vi "Oscilloscope_tests.vi"() -> ()   [LabVIEW 2019]
doc: "This example shows how to configure multiple channels and acquire waveforms from multiple channels."
uses:
  <vilib>/Utility/error.llb/DialogType.ctl
  subVIs/SiPM_Tests_Global_Var.vi
  subVIs/Agilent_lib/Public/Configure/Trigger/Configure Trigger (Edge).vi
  subVIs/Agilent_lib/Agilent 2000 3000 X-Series.lvlib
panel:
  in  "Close Session":bool
  out "Meas Ind":bool
  in  "HP8116A":refnum<visa-resource-name>="GPIB0::16::INSTR" caption="Function Generator HP8116A"
  in  "Power supply Agilent E3631A":refnum<visa-resource-name>="GPIB0::5::INSTR"
  in  "x = y?":bool
  in  "Stop Button 2":bool
  in  "Free Run 2":bool
  in  "Frames to Run":dbl
  in  "Time to Run (s)":dbl
  in  "System Settings":bool
  in  "Load file to display":bool
  in  "Spectrum Only":bool
  in  "Stop Button":bool
  in  "Free Run":bool
  in  "Tab Control":enum32{"Energy Spectrum"}(tab)
  out "XY Graph":T1(graph) caption="Energy Spectrum"
  in  "Coincidence?":bool
  out "en_channels":bool[](array[boolean])
  in  "Trigger Source":T2(ring)
  in  "Input \nCoupling":T3(ring)=enum."DC Coupling"
  in  "Edge \nSlope":enum16{"Pos", "Neg", "Either", "Alt"}(ring)
  in  "Trigger Level (V)":dbl(knob)=0.003 min=-10.0 max=10.0 step=0.01 scale=0.0..5.0
  in  "EN 4":bool=TRUE
  in  "Ch 4 Vertical Scale":dbl(knob)=0.002 min=0.0 max=5.0 step=0.05 scale=0.0..5.0
  in  "CH 4  offset":dbl(knob)=0.006 min=-10.0 max=10.0 step=0.01 scale=0.0..10.0
  in  "Ch3 Vertical Scale":dbl(knob)=0.002 min=0.0 max=5.0 step=0.05 scale=0.0..5.0
  in  "CH 3  offset":dbl(knob)=0.006 min=-10.0 max=10.0 step=0.01 scale=0.0..10.0
  in  "EN 3":bool
  in  "EN 2":bool=TRUE
  in  "Ch 2 Vertical Scale":dbl(knob)=0.002 min=0.0 max=5.0 step=0.05 scale=0.0..5.0
  in  "CH 2  offset":dbl(knob)=0.006 min=-10.0 max=10.0 step=0.01 scale=0.0..10.0
  in  "Ch1 Vertical Scale":dbl(knob)=0.002 min=0.0 max=5.0 step=0.001 scale=0.0..5.0
  in  "CH 1  offset":dbl(knob)=0.006 min=-10.0 max=10.0 step=0.01 scale=0.0..10.0
  in  "EN":bool=TRUE
  in  "Agilent MSO-X 3104A \nOscilloscope":refnum<visa-resource-name>="USB0::0x0957::0x1780::MY56270584::INSTR"
  out "Scope":waveform(dbl)[](graph)
  in  "Impedance":enum16{"1 MOhm", "50 Ohm"}(ring)=enum."50 Ohm"
  in  "Coupling":enum16{"AC", "DC"}(ring)=enum."DC"
  in  "Vertical Setting":enum16{"Vertical Scale", "Vertical Range"}(ring)
  in  "Vertical Range":dbl=40.0
  in  "Time per Division":dbl(knob)=1e-06 scale=0.0..1.0
  in  "Horizontal \nPosition":dbl(knob) scale=0.0..1.0
  in  "Ch1":u8=1 min=1 max=10 step=9
  in  "Ch2":u8=1 min=1 max=10 step=9
  in  "Ch3":u8=1 min=1 max=10 step=9
  in  "Ch4":u8=1 min=1 max=10 step=9
  in  "Bin Min (V)":dbl format="%#_6p"
  in  "Bin Max (V)":dbl=0.026 format="%#_6p"
  out "Pulser":bool
  out "Bias":bool
  out "Power":bool
  out "Scope":bool
  out "Session Log":string
  in  "Read Temperature":bool
  out "Celcius":dbl(slide) scale=0.0..30.0
  in  "Default?":bool=TRUE
  out "Time (s)":dbl format="%.2f"
  in  "Save Results?":bool
  in  "Temperature":string
  in  "Settings Button":bool
  in  "Results Directory":path=path "C:/Users/johnk/Desktop/ESA_Scintillator_Data"
  out "Frames Recorded":i32
  in  "Measurement":string
  in  "File Name":string="1"
  in  "Enable\nVernier":bool
  in  "Enable \nREF \nBNC":bool
  in  "Time Base Type":i32(ring) items=["Main", "Window", "XY", "Roll"]
  # "NCSR  DEMOKRITOS\nInstitute of Nuclear and Particle Physics\nDetectors Instrumentation Laboratory"
  # "CFD Scope Tests"
  # "Record Waveform"
  # "Run Noise Tests"
  # "Probe Attenuation"
  # "RIGOL DG4102 \nFunction Generator"
  # "Histogram Bin"
  # "CH1\n30V/3A"
  # "CH2\n(HV)"
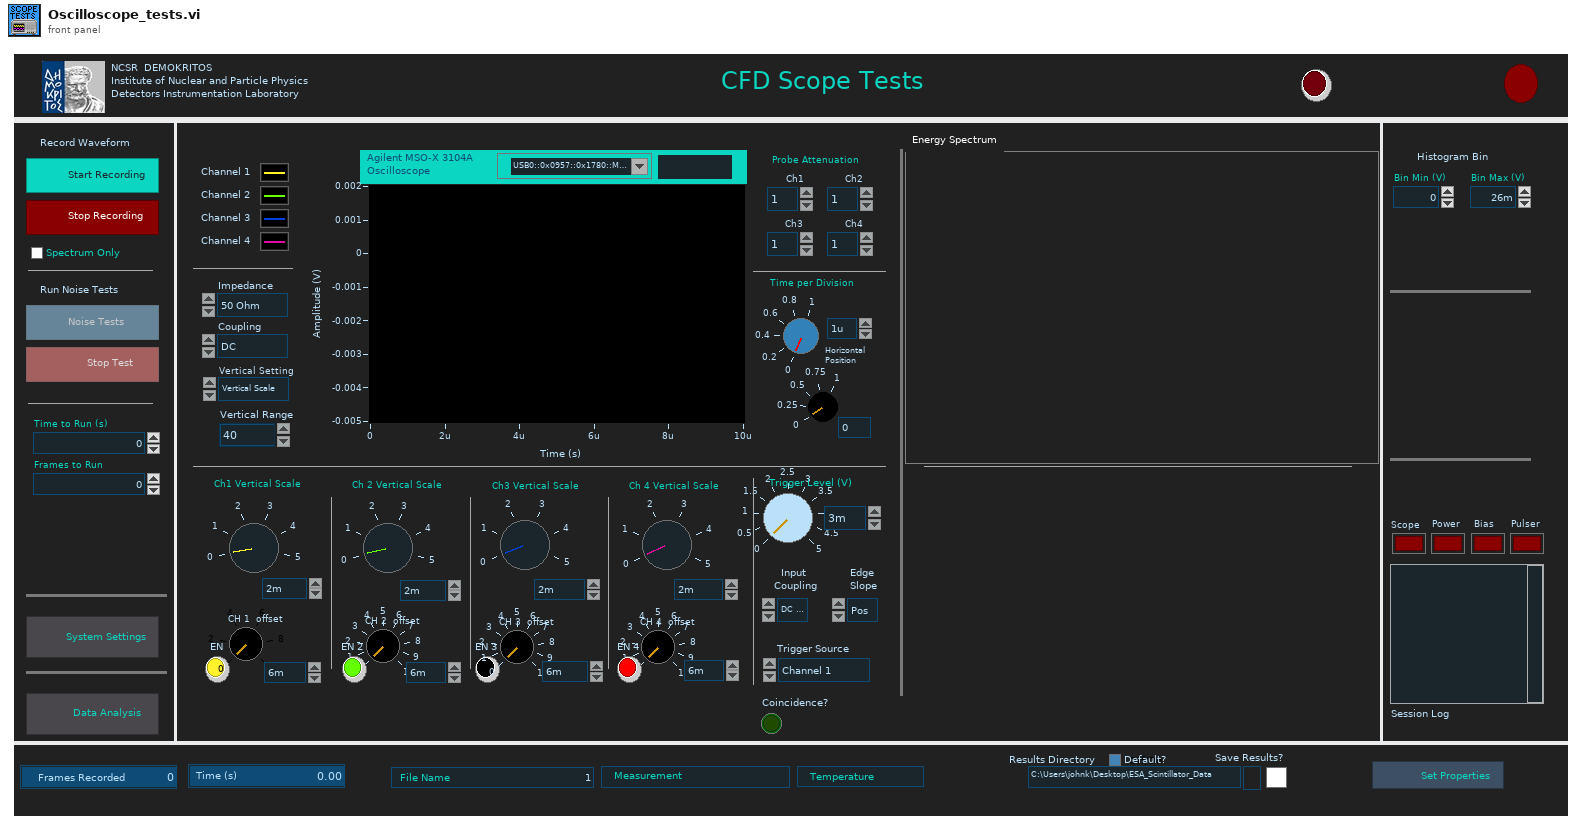
[diagram p1: front panel]
types:
  T1 = cluster{"X Values":dbl[], "Histogram: h(x)":i32[]}[]
  T2 = enum16{"Channel 1", "Channel 2", "Channel 3", "Channel 4", "D0", "D1", "D2", "D3", "D4", "D5", "D6", "D7", "D8", "D9", "D10", "D11", "D12", "D13", "D14", "D15", "External", "Power Line", "Waveform Generator"}
  T3 = enum16{"AC Coupling", "DC Coupling", "Low Frequency Reject"}
  T4 = typedef "DialogType.ctl" = u16
  T5 = cluster{"error":bool, "code":i32, "source":string}
  T6 = enum16{"big-endian, network order", "native, host order", "little-endian"}
  T7 = enum16{"open", "open or create", "create or replace", "create", "open (read-only)"}
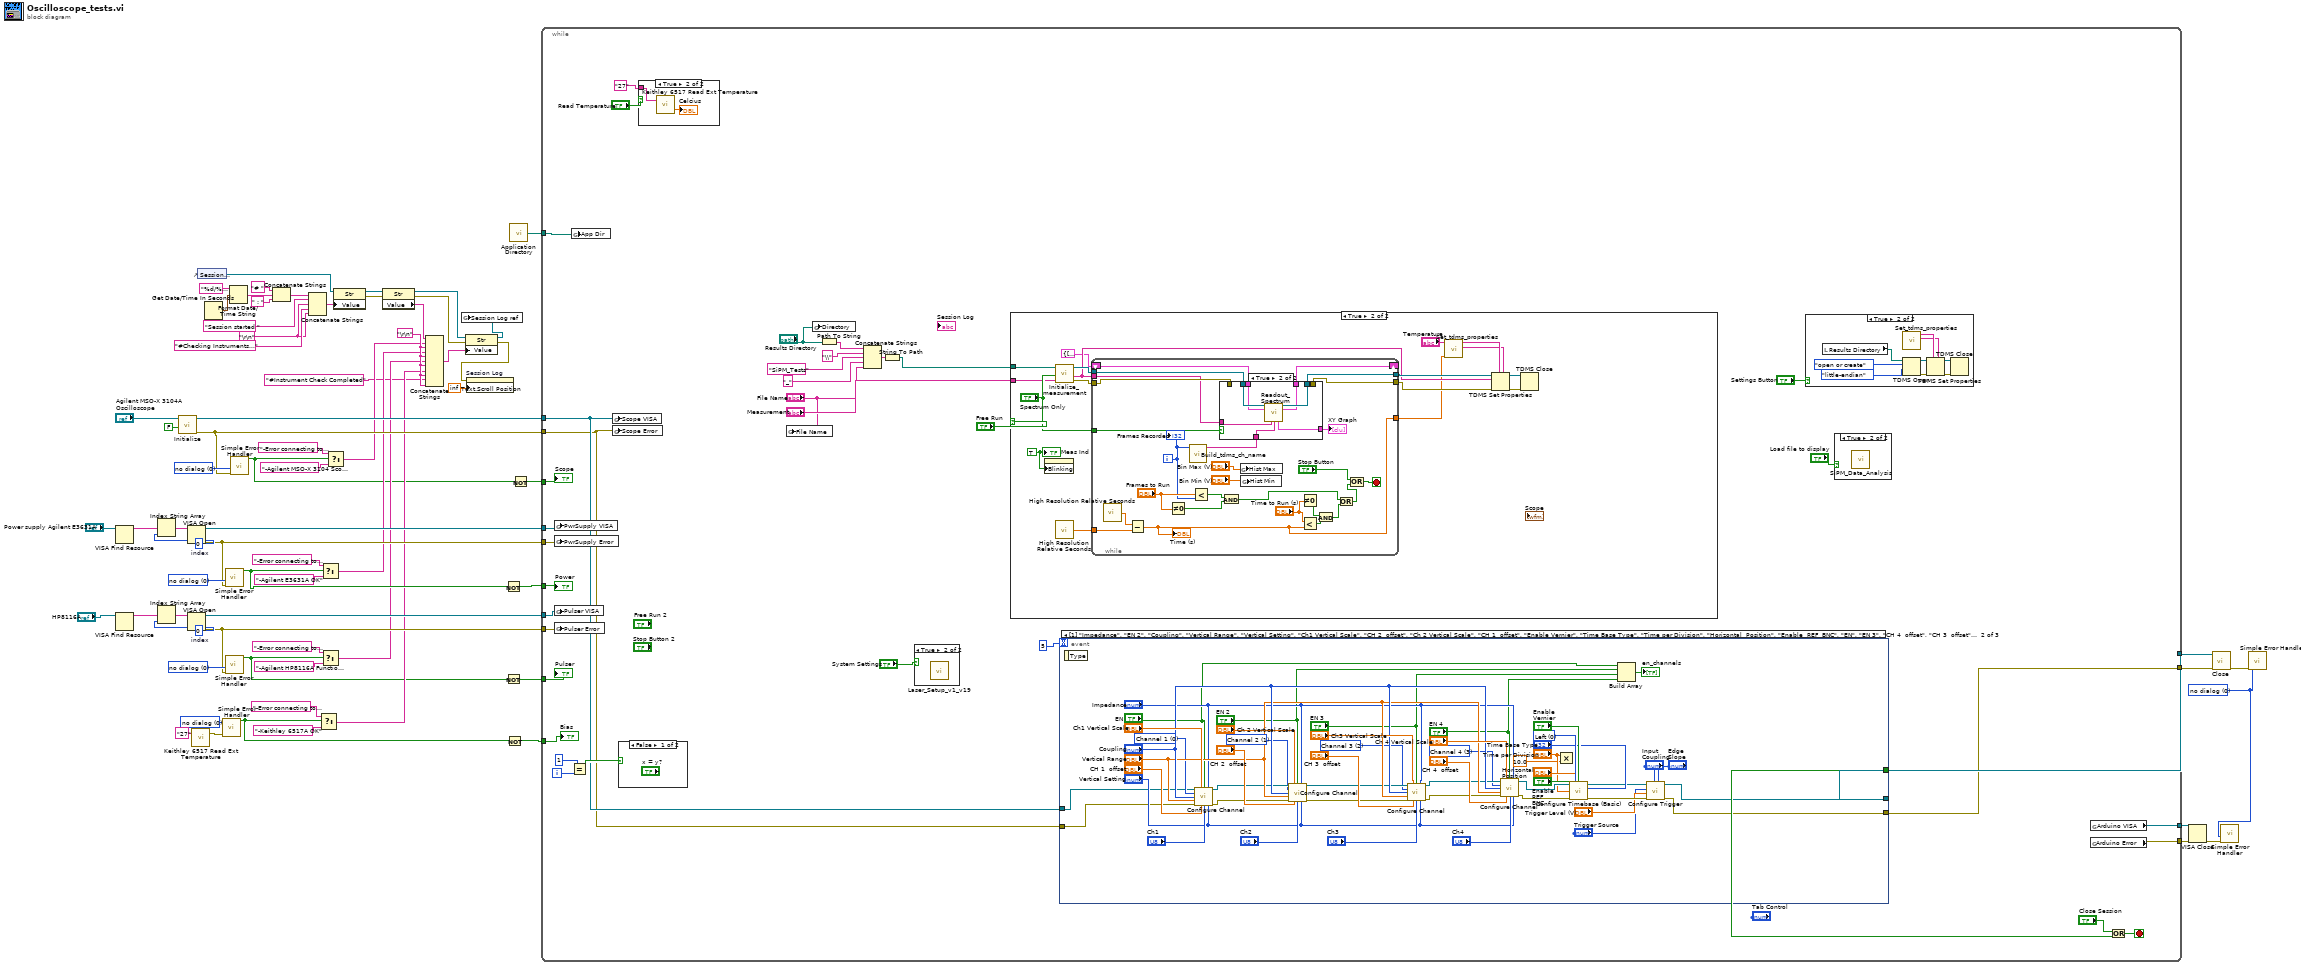
[diagram p0: block diagram]
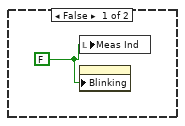
[diagram p4: hidden frame]
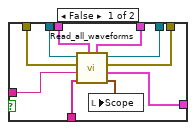
[diagram p5: hidden frame]
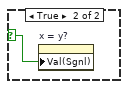
[diagram p6: hidden frame]
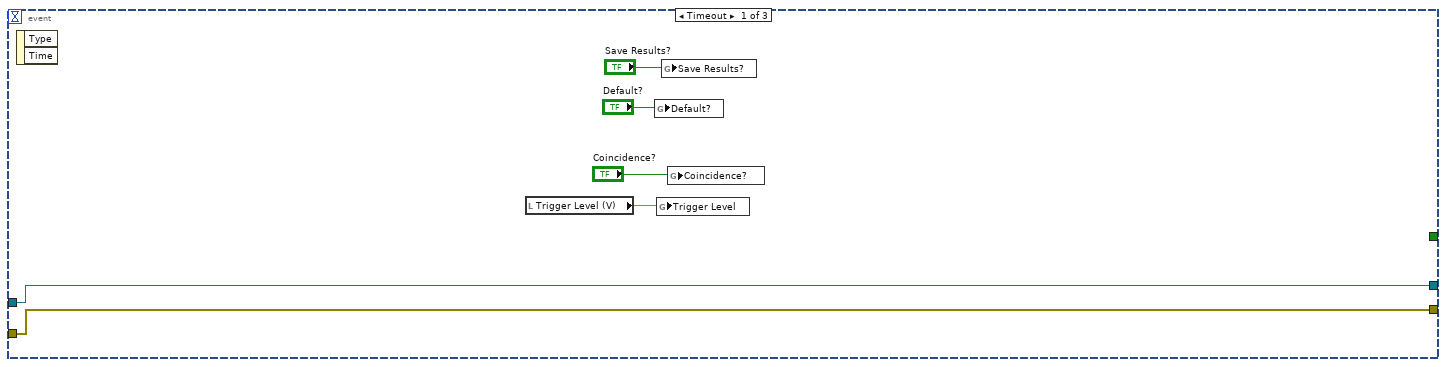
[diagram p9: hidden frame]
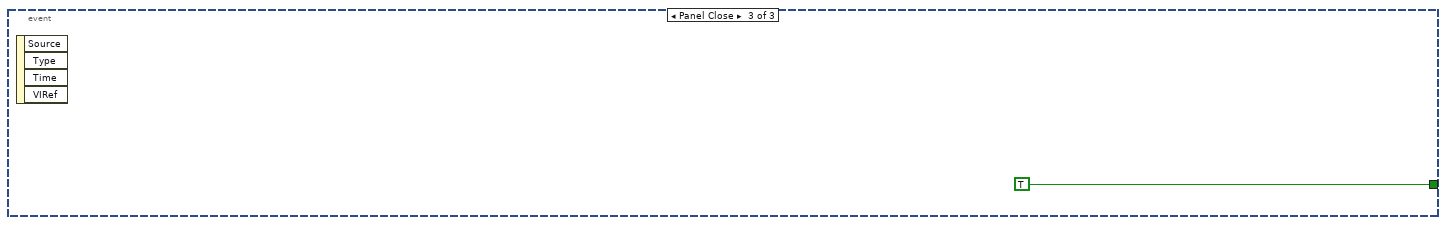
[diagram p10: hidden frame]
diagram:
  w1 = T4 0 items=["no dialog", "OK message", "continue or stop message", "OK message + warnings", "continue/stop + warnings"] ("type of dialog (OK msg:1)")
  w20 = T4 0 items=["no dialog", "OK message", "continue or stop message", "OK message + warnings", "continue/stop + warnings"] ("type of dialog (OK msg:1)")
  w31 = T4 0 items=["no dialog", "OK message", "continue or stop message", "OK message + warnings", "continue/stop + warnings"] ("type of dialog (OK msg:1)")
  w27 = 0  # index
  w36 = T4 0 items=["no dialog", "OK message", "continue or stop message", "OK message + warnings", "continue/stop + warnings"] ("type of dialog (OK msg:1)")
  w42 = 0  # index
  w48 = T4 0 items=["no dialog", "OK message", "continue or stop message", "OK message + warnings", "continue/stop + warnings"] ("type of dialog (OK msg:1)")
  w52 = "\r\n"
  w58 = "\r\n"
  w67 = FALSE ("ID Query (True)")
  n1 = VISA Find Resource(11:"Power supply Agilent E3631A") -> (3:w41:string[])  [unwired: 2 in, 2 out]
  n2 = VISA Find Resource(11:"HP8116A") -> (3:w28:string[])  [unwired: 2 in, 2 out]
  n3 = Index String Array(1:w42, 2:w41) -> (0:w39:string)  [unwired: 1 in]
  n4 = Index String Array(1:w27, 2:w28) -> (0:w29:string)  [unwired: 1 in]
  n5 = call "Initialize.vi"("Reset (True)"=w67, "ID Query (True)"=w67, "VISA resource name"="Agilent MSO-X 3104A \nOscilloscope") -> ("error out"=w47:errorcluster, "VISA resource name out"=w71:refnum<visa-resource-name>)  [unwired: 2 in, 5 out]
  n6 = VISA Open(VISA resource name=w39) -> (VISA resource name=w38:refnum<visa-resource-name>, error out=w35:errorcluster)  [unwired: 4 in]
  n7 = VISA Open(VISA resource name=w29) -> (VISA resource name=w25:refnum<visa-resource-name>, error out=w24:errorcluster)  [unwired: 4 in]
  n8 = call "Keithley 6517 Read Ext Temperature.vi"("GPIB address"="27") -> ("error out"=w21:T5)  [unwired: 1 in, 1 out]
  n9 = control-ref of="Session Log"() -> (w54:refnum<vi>)
  n10 = Get Date/Time In Seconds() -> (seconds since 1Jan1904=w64:timestamp)
  n11 = call <vilib>:"Simple Error Handler.vi"("type of dialog (OK msg:1)"=w20, "error in (no error)"=w21) -> ("error?"=w14:bool)  [unwired: 3 in, 4 out]
  n12 = call <vilib>:"Simple Error Handler.vi"("type of dialog (OK msg:1)"=w36, "error in (no error)"=w35) -> ("error?"=w33:bool)  [unwired: 3 in, 4 out]
  n13 = call <vilib>:"Simple Error Handler.vi"("type of dialog (OK msg:1)"=w31, "error in (no error)"=w24) -> ("error?"=w12:bool)  [unwired: 3 in, 4 out]
  n14 = Format Date/Time String(time format string (%c)="%d/%m/%y_%H:%M:%S", seconds (now)=w64) -> (date/time string=w62:string)  [unwired: 1 in]
  n15 = call <vilib>:"Simple Error Handler.vi"("type of dialog (OK msg:1)"=w48, "error in (no error)"=w47) -> ("error?"=w9:bool)  [unwired: 3 in, 4 out]
  n16 = Concatenate Strings("# " ("string"), w62, " : " ("string")) -> (w61:string)
  n17 = Concatenate Strings(w61, "Session started ", w58, "#Checking Instruments..." ("string"), w58) -> (w57:string)
  n18 = Select(t="-Error connecting to Keithley 6517A" ("Session string"), s=w14, f="-Keithley 6517A OK" ("Session string")) -> (s? t:f=w16:string)
  n19 = Select(t="-Error connecting to Agilent E3631A" ("Session string"), s=w33, f="-Agilent E3631A OK" ("Session string")) -> (s? t:f=w34:string)
  n20 = Select(t="-Error connecting to HP8116A Function Generator" ("Session string"), s=w12, f="-Agilent HP8116A Function Generator OK" ("Session string")) -> (s? t:f=w23:string)
  n21 = Select(t="-Error connecting to Agilent MSO-X3104A Scope" ("Session string"), s=w9, f="-Agilent MSO-X 3104 Scope OK" ("Session string")) -> (s? t:f=w43:string)
  n22 = property on="Property Node" class="Str"(reference=w54, "Value"=w57) -> (reference out=w56:refnum<vi>, error out=w55:errorcluster)  [unwired: 1 in]
  n23 = property on="Property Node" class="Str"(reference=w56, error in=w55) -> (reference out=w50:refnum<vi>, error out=w51:errorcluster, "Value"=w44:string)
  n24 = Concatenate Strings(w44, w43, w52, w34, w52, w23, w52, w16, w52, "#Instrument Check Completed" ("string"), w52) -> (w53:string)
  n25 = property on="Property Node" class="Str"(reference=w50, error in=w51, "Value"=w53) -> (reference out=w49:refnum<vi>, error out=w6:errorcluster)
  n26 = global write "SiPM_Tests_Global_Var.vi" "Session Log ref"(w49) -> ()
  n27 = property on="Session Log" class="Str"(error in=w6, "Text.Scroll Position"=inf) -> ()  [unwired: 1 in, 2 out]
  n28 = Not(x=w33) -> (.not. x?=w32:bool)
  n29 = Not(x=w12) -> (.not. x?=w17:bool)
  n30 = Not(x=w14) -> (.not. x?=w13:bool)
  n31 = call <vilib>:"Application Directory.vi"() -> ("Application Directory"=w2:path)
  n32 = Not(x=w9) -> (.not. x?=w8:bool)
  n33 = while {
    tunnel: w71 -> [w80]
    tunnel: w47 -> [w79]
    tunnel: [w107] -> w70
    tunnel: [w106] -> w69
    tunnel: w38 -> [w84]
    tunnel: w35 -> [w83]
    tunnel: w8 -> [w88]
    tunnel: w32 -> [w87]
    tunnel: w25 -> [w82]
    tunnel: w24 -> [w81]
    tunnel: w17 -> [w86]
    tunnel: w13 -> [w85]
    tunnel: [w77] -> w4
    tunnel: [w76] -> w3
    tunnel: w2 -> [w73]
    i -> [w95]
    stop <- w100 stop-if-true
    n34 = global write "SiPM_Tests_Global_Var.vi" "PwrSupply VISA"(w84) -> ()
    n35 = global write "SiPM_Tests_Global_Var.vi" "PwrSupply Error"(w83) -> ()
    n36 = global write "SiPM_Tests_Global_Var.vi" "Pulser VISA"(w82) -> ()
    n37 = global write "SiPM_Tests_Global_Var.vi" "Pulser Error"(w81) -> ()
    n38 = Equal?(x=1, y=w95) -> (x = y?=w93:bool)
    n39 = global write "SiPM_Tests_Global_Var.vi" "App Dir"(w73) -> ()
    n40 = global write "SiPM_Tests_Global_Var.vi" "Scope VISA"(w80) -> ()
    n41 = global write "SiPM_Tests_Global_Var.vi" "Scope Error"(w79) -> ()
    n42 = case shown="False" w93 {
      selector: w93 -> [_ w181]
      frame False {
      }
      frame True {
        n43 = property on="x = y?" class="Bool (strict)"("Val(Sgnl)"=w181) -> ()  [unwired: 2 in, 2 out]
      }
    }
    n44 = case shown="True" "Read Temperature" {
      tunnel: "27" ("GPIB address") -> [_ w183]
      frame False {
      }
      frame True {
        n45 = call "Keithley 6517 Read Ext Temperature.vi"("GPIB address"=w183) -> ("External Temperature"=→"Celcius":dbl)  [unwired: 1 in, 1 out]
      }
    }
    n46 = global write "SiPM_Tests_Global_Var.vi" "File Name"("File Name") -> ()
    n47 = global write "SiPM_Tests_Global_Var.vi" "Directory"("Results Directory") -> ()
    n48 = Path To String(path="Results Directory") -> (string=w102:string)
    n49 = Concatenate Strings(w102, "\\" ("string"), "SiPM_Tests", "_", "File Name") -> (w101:string)
    n50 = String To Path(string=w101) -> (path=w92:path)
    n51 = case shown="True" "System Settings" {
      frame False {
      }
      frame True {
        n52 = call "Laser_Setup_v1_v19.vi"() -> ()  [unwired: 12 in]
      }
    }
    n53 = case shown="True" "Free Run" {
      tunnel: w92 -> [_ w127]
      tunnel: "Measurement" -> [_ w128]
      frame False {
        w119 = FALSE ("Meas Ind")
        n54 = local write "Meas Ind"(w119) -> ()
        n55 = property on="Meas Ind" class="Bool (strict)"("Blinking"=w119) -> ()  [unwired: 2 in, 2 out]
      }
      frame True {
        w134 = TRUE ("Measurements  ON")
        n56 = property on="Meas Ind" class="Bool (strict)"("Blinking"=w134) -> ()  [unwired: 2 in, 2 out]
        n57 = call "Initialize_measurement.vi"("Measurement"=w128, "Spectrum Only?"="Spectrum Only", "file path"=w127) -> ("error out"=w130:errorcluster, "Group Name"=w122:string, "tdms file out"=w131:refnum<k34>)  [unwired: 6 in]
        n58 = call <vilib>:"High Resolution Relative Seconds.vi"() -> ("relative seconds"=w126:dbl)
        n59 = while {
          tunnel: w131 -> [w163]
          tunnel: w130 -> [w162]
          tunnel: "Spectrum Only" -> [w159]
          tunnel: [w161] -> w133
          tunnel: [w160] -> w132
          tunnel: w122 -> [w158]
          tunnel: w126 -> [w155]
          shift-right: [w149] -> _
          shift-left: cluster{dbl[], dbl[], dbl[], dbl[]} {[], [], [], []} ("Peak_data_in") -> [w150]
          tunnel: [w137] -> w121
          i -> [w145]
          stop <- w140 stop-if-true
          n60 = call <vilib>:"High Resolution Relative Seconds.vi"() -> ("relative seconds"=w156:dbl)
          n61 = Subtract(x=w156, y=w155) -> (x-y=w137:dbl)
          "Time (s)" <- w137
          n62 = Not Equal To 0?(x="Frames to Run") -> (x != 0?=w143:bool)
          n63 = call "Build_tdms_ch_name.vi"("Frame_nb"=w145) -> ("Channel_name"=w148:string[])  [unwired: 10 in]
          n64 = Less?(x="Frames to Run", y=w145) -> (x < y?=w144:bool)
          n65 = case shown="True" w159 {
            tunnel: w163 -> [w173 w180]
            tunnel: w162 -> [w172 _]
            tunnel: [w171 w179] -> w161
            tunnel: [w170 _] -> w160
            tunnel: w158 -> [w168 w174]
            tunnel: w148 -> [w167 w175]
            tunnel: [w166 w176] -> w138
            tunnel: w150 -> [w165 w178]
            tunnel: [w164 w177] -> w149
            frame False {
              n66 = call "Read_all_waveforms.vi"("Peak_data_in"=w165, "Channel names"=w167, "Group name"=w168, "error in"=w172, "tdms file in"=w173) -> ("Waveforms"=w169:waveform(dbl)[], "Spectrum"=w166:T1, "error out"=w170:errorcluster, "tdms file out"=w171:refnum<k34>, "Peak_data_out"=w164:cluster{dbl[], dbl[], dbl[], dbl[]})  [unwired: 2 in]
              n67 = local write "Scope"(w169) -> ()
            }
            frame True {
              n68 = call "Readout_Spectrum.vi"("tdms file in"=w180, "Ch_in"=w178, "group name"=w174, "channel names"=w175) -> ("tdms file out"=w179:refnum<k34>, "Ch_out"=w177:cluster{dbl[], dbl[], dbl[], dbl[]}, "Spectrum_out"=w176:T1)  [unwired: 9 in]
            }
          }
          "XY Graph" <- w138
          n69 = And(x=w144, y=w143) -> (x .and. y?=w142:bool)
          n70 = global write "SiPM_Tests_Global_Var.vi" "Hist Max"("Bin Max (V)") -> ()
          n71 = global write "SiPM_Tests_Global_Var.vi" "Hist Min"("Bin Min (V)") -> ()
          n72 = Not Equal To 0?(x="Time to Run (s)") -> (x != 0?=w153:bool)
          n73 = Less?(x="Time to Run (s)", y=w137) -> (x < y?=w154:bool)
          n74 = And(x=w153, y=w154) -> (x .and. y?=w151:bool)
          n75 = Or(x=w142, y=w151) -> (x .or. y?=w141:bool)
          n76 = Or(x="Stop Button", y=w141) -> (x .or. y?=w140:bool)
          "Frames Recorded" <- w145
        }
        n77 = call "Set_tdms_properties.vi"("Measurement Duration(s)"=w121, "Temperature"="Temperature") -> ("Property Values"=w123:string[], "property names"=w124:string[])  [unwired: 8 in]
        n78 = TDMS Set Properties(5:w123, 7:w124, 8:w132, 10:w122, 11:w133) -> (0:w135:errorcluster, 3:w136:refnum<k34>)  [unwired: 1 in, 2 out]
        n79 = TDMS Close(8:w135, 11:w136) -> ()  [unwired: 2 out]
        "Meas Ind" <- w134
      }
    }
    n80 = event shown="[1] \"Impedance\", \"EN 2\", \"Coupling\", \"Vertical Range\", \"Vertical Setting\", \"Ch1 Vertical Scale\", \"CH 2  offset\", \"Ch 2 Vertical Scale\", \"CH 1  offset\", \"Enable Vernier\", \"Time Base Type\", \"Time per Division\", \"Horizontal  Position\", \"Enable  REF  BNC\", \"EN\", \"EN 3\", \"CH 4  offset\", \"CH 3  offset\", \"Ch 4 Vertical Scale\", \"EN 4\", \"Ch3 Vertical Scale\", \"Trigger Level (V)\", \"Input  Coupling\", \"x = y?\": Value Change" {
      selector: _ -> [_ _ _]
      dyn-events: _ -> [_ _ _]
      timeout: 5 -> [_ _ _]
      tunnel: w80 -> [w189 w207 _]
      tunnel: w79 -> [w188 w206 _]
      tunnel: [w189 w204 _] -> w107
      tunnel: [w188 w202 _] -> w106
      tunnel: [_ _ TRUE ("y")] -> w98
      event Timeout {
        n81 = event-data() -> ()  [unwired: 1 in, 2 out]
        n82 = local read "Trigger Level (V)"() -> (w184:dbl)
        n83 = global write "SiPM_Tests_Global_Var.vi" "Default?"("Default?") -> ()
        n84 = global write "SiPM_Tests_Global_Var.vi" "Trigger Level"(w184) -> ()
        n85 = global write "SiPM_Tests_Global_Var.vi" "Save Results?"("Save Results?") -> ()
        n86 = global write "SiPM_Tests_Global_Var.vi" "Coincidence?"("Coincidence?") -> ()
      }
      event "Impedance", "EN 2", "Coupling", "Vertical Range", "Vertical Setting", "Ch1 Vertical Scale", "CH 2  offset", "Ch 2 Vertical Scale", "CH 1  offset", "Enable\nVernier", "Time Base Type", "Time per Division", "Horizontal \nPosition", "Enable \nREF \nBNC", "EN", "EN 3", "CH 4  offset", "CH 3  offset", "Ch 4 Vertical Scale", "EN 4", "Ch3 Vertical Scale", "Trigger Level (V)", "Input \nCoupling", "x = y?": Value Change {
        w231 = 0 items=["Left", "Center", "Right"] ("Reference")
        w208 = 3 items=["Channel 1", "Channel 2", "Channel 3", "Channel 4"] ("Channel Name (0: Channel 1)")
        w209 = 2 items=["Channel 1", "Channel 2", "Channel 3", "Channel 4"] ("Channel Name (0: Channel 1)")
        w210 = 1 items=["Channel 1", "Channel 2", "Channel 3", "Channel 4"] ("Channel Name (0: Channel 1)")
        w211 = 0 items=["Channel 1", "Channel 2", "Channel 3", "Channel 4"] ("Channel Name (0: Channel 1)")
        n87 = event-data() -> ()  [unwired: 1 in, 1 out]
        n88 = call "Configure Channel.vi"("VISA resource name"=w207, "Vertical Scale (5.0 V)"="Ch1 Vertical Scale", "Enable Channel (T: Enable)"="EN", "Impedance (0: 1 MOhm)"="Impedance", "Channel Name (0: Channel 1)"=w211, "Coupling (1: DC)"="Coupling", "Vertical Range (40.0 V)"="Vertical Range", "error in (no error)"=w206, "Vertical Offset (0.0)"="CH 1  offset", "Probe Attenuation (1.0)"="Ch1", "Vertical Setting (1: Vertical Range)"="Vertical Setting") -> ("VISA resource name out"=w219:refnum<visa-resource-name>, "error out"=w218:errorcluster)  [unwired: 3 out]
        n89 = call "Configure Channel.vi"("VISA resource name"=w219, "Vertical Scale (5.0 V)"="Ch 2 Vertical Scale", "Enable Channel (T: Enable)"="EN 2", "Impedance (0: 1 MOhm)"="Impedance", "Channel Name (0: Channel 1)"=w210, "Coupling (1: DC)"="Coupling", "Vertical Range (40.0 V)"="Vertical Range", "error in (no error)"=w218, "Vertical Offset (0.0)"="CH 2  offset", "Probe Attenuation (1.0)"="Ch2", "Vertical Setting (1: Vertical Range)"="Vertical Setting") -> ("VISA resource name out"=w217:refnum<visa-resource-name>, "error out"=w216:errorcluster)  [unwired: 3 out]
        n90 = call "Configure Channel.vi"("VISA resource name"=w217, "Vertical Scale (5.0 V)"="Ch3 Vertical Scale", "Enable Channel (T: Enable)"="EN 3", "Impedance (0: 1 MOhm)"="Impedance", "Channel Name (0: Channel 1)"=w209, "Coupling (1: DC)"="Coupling", "Vertical Range (40.0 V)"="Vertical Range", "error in (no error)"=w216, "Vertical Offset (0.0)"="CH 3  offset", "Probe Attenuation (1.0)"="Ch3", "Vertical Setting (1: Vertical Range)"="Vertical Setting") -> ("VISA resource name out"=w215:refnum<visa-resource-name>, "error out"=w214:errorcluster)  [unwired: 3 out]
        n91 = call "Configure Channel.vi"("VISA resource name"=w215, "Vertical Scale (5.0 V)"="Ch 4 Vertical Scale", "Enable Channel (T: Enable)"="EN 4", "Impedance (0: 1 MOhm)"="Impedance", "Channel Name (0: Channel 1)"=w208, "Coupling (1: DC)"="Coupling", "Vertical Range (40.0 V)"="Vertical Range", "error in (no error)"=w214, "Vertical Offset (0.0)"="CH 4  offset", "Probe Attenuation (1.0)"="Ch4", "Vertical Setting (1: Vertical Range)"="Vertical Setting") -> ("VISA resource name out"=w213:refnum<visa-resource-name>, "error out"=w212:errorcluster)  [unwired: 3 out]
        n92 = Multiply(x="Time per Division", y=10.0) -> ()  [unwired: 1 out]
        n93 = call "Configure Timebase (Basic).vi"("VISA resource name"=w213, "Reference (1: Center)"=w231, "Enable Vernier (F: Disable)"="Enable\nVernier", "Time Base Type (0: Main)"="Time Base Type", "Scale (50 s/div)"="Time per Division", "error in (no error)"=w212, "Position (0.0)"="Horizontal \nPosition", "Enable REF BNC (F: Disable)"="Enable \nREF \nBNC") -> ("VISA resource name out"=w205:refnum<visa-resource-name>, "error out"=w203:errorcluster)  [unwired: 1 in, 5 out]
        n94 = Build Array("EN", "EN 2", "EN 3", "EN 4") -> (→"en_channels":bool[])
        n95 = call-poly "Configure Trigger.vi"("Edge Slope (0: Positive)"="Edge \nSlope", "Input Coupling (0: AC Coupling)"="Input \nCoupling", "error in (no error)"=w203, "Trigger Level (0 V)"="Trigger Level (V)", "Trigger Source (0: Channel 1)"="Trigger Source", "VISA resource name"=w205) -> ("error out"=w202:errorcluster, "VISA resource name out"=w204:refnum<visa-resource-name>)  [unwired: 4 in]
      }
      event Panel Close {
        n96 = event-data() -> ()  [unwired: 1 in, 4 out]
      }
    }
    n97 = case shown="True" "Settings Button" {
      frame False {
      }
      frame True {
        n98 = local read "Results Directory"() -> (w110:path)
        n99 = call "Set_tdms_properties.vi"() -> ("Property Values"=w111:string[], "property names"=w112:string[])  [unwired: 10 in]
        n100 = TDMS Open(9:T6."little-endian" ("byte order (2:little-endian)"), 10:T7."open or create" ("operation (0:open)"), 11:w110) -> (0:w113:errorcluster, 3:w116:refnum<k34>)  [unwired: 4 in]
        n101 = TDMS Set Properties(5:w111, 7:w112, 8:w113, 11:w116) -> (0:w114:errorcluster, 3:w115:refnum<k34>)  [unwired: 2 in, 2 out]
        n102 = TDMS Close(8:w114, 11:w115) -> ()  [unwired: 2 out]
      }
    }
    n103 = case shown="True" "Load file to display" {
      frame False {
      }
      frame True {
        n104 = call "SiPM_Data_Analysis.vi"() -> ()  [unwired: 12 in]
      }
    }
    n105 = global read "SiPM_Tests_Global_Var.vi" "Arduino Error"() -> (w76:errorcluster)
    n106 = global read "SiPM_Tests_Global_Var.vi" "Arduino VISA"() -> (w77:refnum<visa-resource-name>)
    n107 = Or(x="Close Session", y=w98) -> (x .or. y?=w100:bool)
    "Scope" <- w88
    "Power" <- w87
    "Bias" <- w85
    "Pulser" <- w86
  }
  n108 = VISA Close(VISA resource name=w4, error in (no error)=w3) -> (error out=w5:errorcluster)
  n109 = call "Close.vi"("error in (no error)"=w69, "VISA resource name"=w70) -> ("error out"=w72:errorcluster)  [unwired: 9 out]
  n110 = call <vilib>:"Simple Error Handler.vi"("type of dialog (OK msg:1)"=w1, "error in (no error)"=w5) -> ()  [unwired: 8 out]
  n111 = call <vilib>:"Simple Error Handler.vi"("type of dialog (OK msg:1)"=w1, "error in (no error)"=w72) -> ()  [unwired: 8 out]
